vi "Setup TestRunner ClassInstance.vi"(5 "Interactive (T)":bool=TRUE, 7 "Verbose (F)":bool, 8 "error in (no error)":errorcluster, 9 "Test Report":refnum<class "Test Report.lvclass">, 10 "Instance":refnum<class>, 11 "Test Runner.Class in":refnum<class "Test Runner.Class.lvclass">) -> (0 "error out":errorcluster, 3 "Test Runner.Class out":refnum<class "Test Runner.Class.lvclass">)   [LabVIEW 2013, in "Caraya.lvlib" / "Test Runner.Class.lvclass"]
uses:
  Test Runner.Class.lvclass
  Test Report/Test Report.lvclass
  Test Runner/Test Runner.lvclass/Test Runner.ctl
  Test Runner.Class.lvclass/Test Runner.Class.ctl
  Test Runner/Test Runner.lvclass
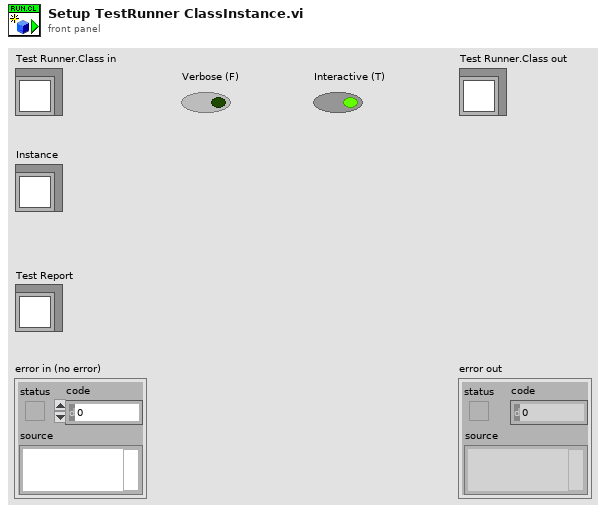
[diagram p1: front panel]
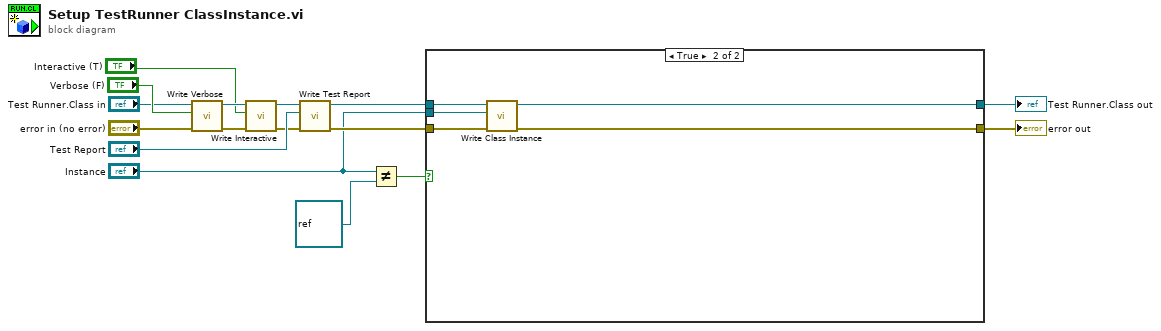
[diagram p0: block diagram]
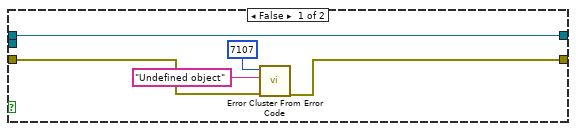
[diagram p2: hidden frame]
diagram:
  n1 = call "Write Verbose.vi"("Verbose"="Verbose (F)", "Test Runner in"="Test Runner.Class in") -> ("Test Runner out"=w8:refnum<class "Test Runner.Class.lvclass">)  [unwired: 9 in]
  n2 = call "Write Interactive.vi"("Interactive"="Interactive (T)", "Test Runner in"=w8) -> ("Test Runner out"=w5:refnum<class "Test Runner.Class.lvclass">)  [unwired: 9 in]
  n3 = call "Write Test Report.vi"("Test Report"="Test Report", "Test Runner in"=w5) -> ("Test Runner out"=w12:refnum<class "Test Runner.Class.lvclass">)  [unwired: 9 in]
  n4 = Not Equal?(x="Instance", y=refnum<class> refnum) -> (x != y?=w1:bool)
  n5 = case shown="True" w1 {
    tunnel: w12 -> [w14 w23]
    tunnel: "error in (no error)" -> [w16 w22]
    tunnel: [w14 w19] -> w11
    tunnel: [w15 w20] -> w10
    tunnel: "Instance" -> [_ w21]
    frame False {
      n6 = call <vilib>:"Error Cluster From Error Code.vi"("error in (no error)"=w16, "error message (\"\")"="Undefined object" ("error message (\"\")"), "error code (0)"=7107) -> ("error out"=w15:errorcluster)  [unwired: 6 in]
    }
    frame True {
      n7 = call "Write Class Instance.vi"("error in (no error)"=w22, "Instance"=w21, "Test Runner.Project in"=w23) -> ("error out"=w20:errorcluster, "Test Runner.Project out"=w19:refnum<class "Test Runner.Class.lvclass">)  [unwired: 7 in]
    }
  }
  "error out" <- w10
  "Test Runner.Class out" <- w11
